vi "Text_Receiver.vi"() -> ()   [LabVIEW 2013]
uses:
  NetHackrf.dll
  <vilib>/addons/Modulation/niDMT.lvlib
panel:
  out "Symbol Rate\n[symbols/sec]":dbl=25000.0 format="%#.6p"
  in  "synchronization parameters":T1={"expected sync location (symbols)"=-1, "sync sequence"=[], "sync location uncertainty (symbols)"=0, "sync indent (symbols)"=0} {"sync sequence" format="%.2f"}
  in  "stop":bool
  in  "Tab Control":T2(tab)=enum."Rx Display"
  in  "Acquisition Duration [sec]":dbl=0.04 format="%#.6p"
  in  "Choose a PSK \nFormat":T3(tab)=enum."QPSK" caption="PSK"
  in  "BPSK System Parameters":T4={"Samples per Symbol"=8, "symbol map"=[], "Differential PSK"=enum."disable", "PSK type"=0} {"PSK type" items=["normal", "shifted", "offset"]; "symbol map" format="%.3f"}
  in  "QPSK System Parameters":T4={"Samples per Symbol"=8, "symbol map"=[], "Differential PSK"=enum."disable", "PSK type"=0} {"PSK type" items=["normal", "shifted", "offset"]; "symbol map" format="%.3f"}
  in  "pi/4 DQPSK System Parameters":T4={"Samples per Symbol"=8, "symbol map"=[], "Differential PSK"=enum."enable", "PSK type"=1} {"PSK type" items=["normal", "shifted", "offset"]; "symbol map" format="%.3f"}
  in  "OQPSK System Parameters":T4={"Samples per Symbol"=8, "symbol map"=[], "Differential PSK"=enum."disable", "PSK type"=2} {"PSK type" items=["normal", "shifted", "offset"]; "symbol map" format="%.3f"}
  in  "8-PSK System Parameters":T4={"Samples per Symbol"=8, "symbol map"=[], "Differential PSK"=enum."disable", "PSK type"=0} {"PSK type" items=["normal", "shifted", "offset"]; "symbol map" format="%.3f"}
  in  "16-PSK System Parameters":T4={"Samples per Symbol"=8, "symbol map"=[], "Differential PSK"=enum."disable", "PSK type"=0} {"PSK type" items=["normal", "shifted", "offset"]; "symbol map" format="%.3f"}
  in  "M":i32=4 min=2 step=2
  in  "Custom System Parameters":T4={"Samples per Symbol"=8, "symbol map"=[], "Differential PSK"=enum."disable", "PSK type"=0} {"PSK type" items=["normal", "shifted", "offset"]; "symbol map" format="%.3f"}
  in  "filter parameters":T5={"Alpha"=0.5, "Filter Length"=6, "TX Filter"=enum."Root Raised Cos"} caption="Matching Filter Parameters" {"Alpha" format="%.2f"}
  in  "PN Sequence Order for Sync":i32=31
  in  "Packet Parameters":T6={"Guard Bits "=30, "Sync Bits"=20, "Message Bits"=128, "Number of Packets \nto Expect"=46}
  out "Recovered Message":string
  out "Received Signal (Raw)":dbl[](graph)
  out "Constellation Graph":T7(graph)
  out "Sync Found":bool
  out "Correct Packets Rx":i16
  in  "Continuous Acquire?":bool
  out "Singal & Noise Power":cluster{"signal_power":dbl, "noise_power":dbl}={"signal_power"=1.4546950663593878e-09, "noise_power"=2.571229598792933e-12}
  out "error out":errorcluster={"status"=FALSE, "code"=1074118647, "source"="niUSRP Fetch Rx Data (CDB Cluster).vi<ERR>Overflow: an internal receive buffer has filled before the data could be returned.  Consider reducing the IQ rate, increasing the Fetch rate, or increasing the number of samples per Fetch."}
  out "Cumulative Packets Recovered":i16(graph)
  out "Signal and Noise Power Tracking":cluster{"total_power":dbl, "noise_power":dbl}(graph)={"total_power"=1.4546950663593878e-09, "noise_power"=2.571229598792933e-12}
  # "Packet Receiver"
  # "Continuous Acquire 设置为TRUE，Stop才有用"
  # "Guard\nBand"
  # "Sync\nSeq"
  # "Packet\nNumber"
  # "Pad\nData"
  # "Blank\nFrame"
  # "Data"
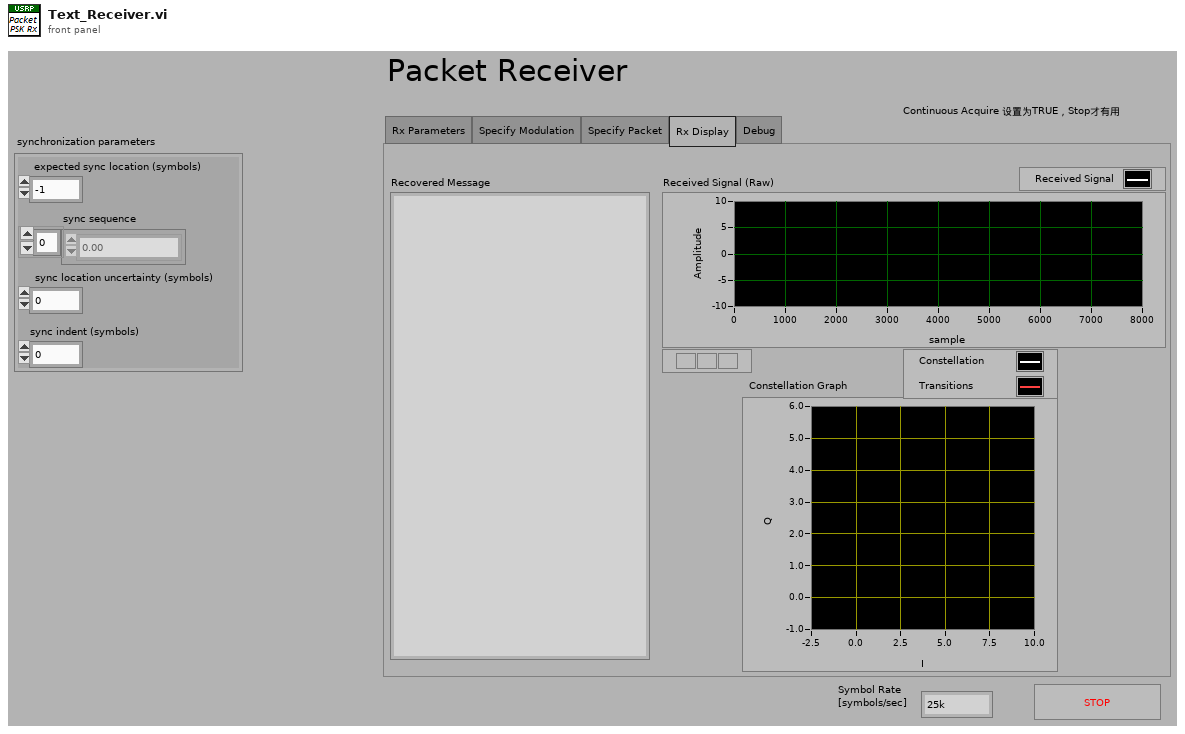
[diagram p1: front panel]
types:
  T1 = cluster{"expected sync location (symbols)":i32, "sync sequence":cdb[], "sync location uncertainty (symbols)":i32, "sync indent (symbols)":i32}
  T2 = enum32{"Rx Parameters", "Specify Modulation", "Specify Packet", "Rx Display", "Debug"}
  T3 = enum32{"BPSK", "QPSK", "pi/4DQPSK", "OQPSK", "8-PSK", "16-PSK", "Custom"}
  T4 = cluster{"Samples per Symbol":i32, "symbol map":cdb[], "Differential PSK":enum16{"disable", "enable"}, "PSK type":u16}
  T5 = cluster{"Alpha":dbl, "Filter Length":i32, "TX Filter":enum16{"none", "Raised Cosine", "Root Raised Cos", "Gaussian"}}
  T6 = cluster{"Guard Bits ":i32, "Sync Bits":i32, "Message Bits":i32, "Number of Packets \nto Expect":i32}
  T7 = cluster{"Decimated Array":dbl[], "Decimated Array":dbl[]}[]
  T8 = cluster{"Packet Array":i32[][], "IP Array of Pkt Nums Received  ":bool[]}
  T9 = cluster{"bit stream ":i8[][], "Sync Valid?":bool[], "Decoded Pkt Numbers":u32[], "Enable?":bool}
  T10 = cluster{"packet_arr":cdb[][], "Packets Valid?":bool}
  T11 = cluster{"PSK type":u16, "Samples per Symbol":i32, "Differential PSK":enum16{"disable", "enable"}, "M":i32}
  T12 = cluster{"PSK system parameters":cluster{"samples per symbol (16)":i32, "symbol map":cdb[], "differential PSK":enum16{"disable", "enable"}, "PSK type":u16}, "pulse shaping filter coefficients":dbl[], "matched filter coefficients":dbl[], "synchronization parameters":cluster{"expected sync location (symbols)":i32, "sync sequence":cdb[], "sync location uncertainty (symbols)":i32, "sync indent (symbols)":i32}, "Sync Bits":i8[]}
  T13 = typedef "niAMT.lvlib/Complex Data Waveform.ctl" = cluster{"t0":dbl, "dt":dbl, "Y":cdb[]}
  T14 = cluster{"constellation":dbl[], "oversampled data":dbl[]}[]
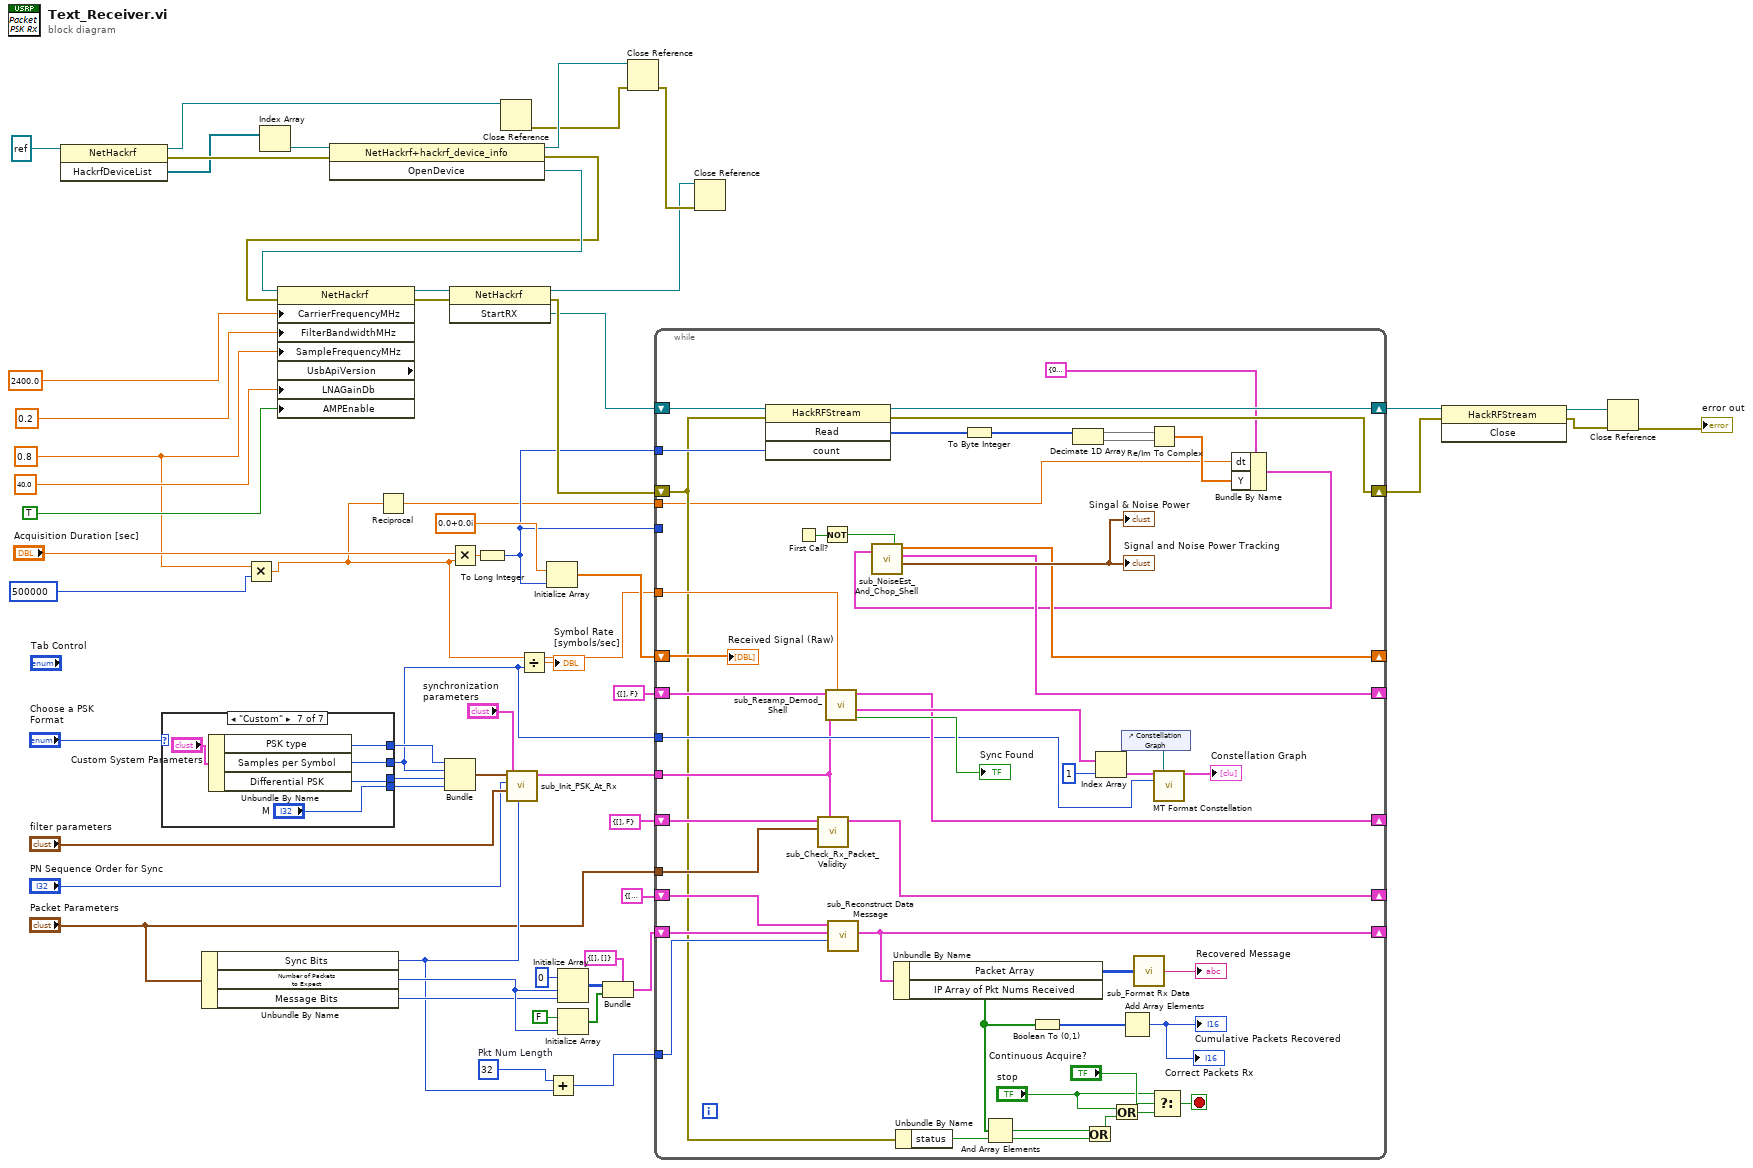
[diagram p0: block diagram]
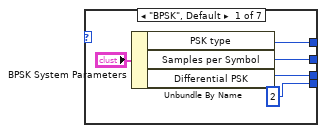
[diagram p2: hidden frame]
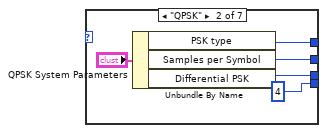
[diagram p3: hidden frame]
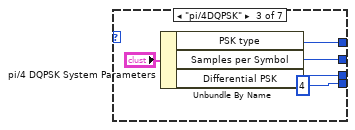
[diagram p4: hidden frame]
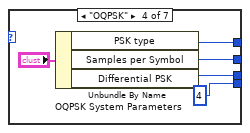
[diagram p5: hidden frame]
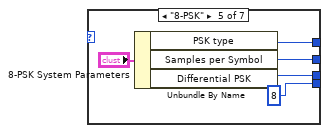
[diagram p6: hidden frame]
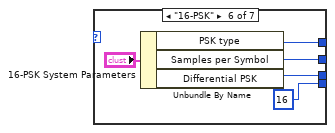
[diagram p7: hidden frame]
diagram:
  w13 = 0.8 ("SampleFrequencyMHz")
  w46 = 32  # Pkt Num Length
  n1 = invoke class="NetHackrf" method="HackrfDeviceList"(reference=refnum<k24> refnum) -> (reference out=w20:refnum<k24>, error out=w29:errorcluster, "HackrfDeviceList"=w27:refnum<k24>[])  [unwired: 2 in]
  n2 = case shown="\"Custom\"" "Choose a PSK \nFormat" {
    tunnel: [w62 w68 w73 w78 w83 w89 w92] -> w43
    tunnel: [w63 w66 w72 w77 w82 w88 w93] -> w52
    tunnel: [2 ("M-PSK (4)") 4 ("M-PSK (4)") 4 ("M-PSK (4)") 4 ("M-PSK (4)") 8 ("M-PSK (4)") 16 ("M-PSK (4)") "M"] -> w51
    tunnel: [w64 w67 w71 w76 w84 w87 w94] -> w53
    frame "BPSK", Default {
      n3 = Unbundle By Name("BPSK System Parameters") -> ("PSK type"=w64:u16, "Samples per Symbol"=w62:i32, "Differential PSK"=w63:enum16{"disable", "enable"})
    }
    frame "QPSK" {
      n4 = Unbundle By Name("QPSK System Parameters") -> ("PSK type"=w67:u16, "Samples per Symbol"=w68:i32, "Differential PSK"=w66:enum16{"disable", "enable"})
    }
    frame "pi/4DQPSK" {
      n5 = Unbundle By Name("pi/4 DQPSK System Parameters") -> ("PSK type"=w71:u16, "Samples per Symbol"=w73:i32, "Differential PSK"=w72:enum16{"disable", "enable"})
    }
    frame "OQPSK" {
      n6 = Unbundle By Name("OQPSK System Parameters") -> ("PSK type"=w76:u16, "Samples per Symbol"=w78:i32, "Differential PSK"=w77:enum16{"disable", "enable"})
    }
    frame "8-PSK" {
      n7 = Unbundle By Name("8-PSK System Parameters") -> ("PSK type"=w84:u16, "Samples per Symbol"=w83:i32, "Differential PSK"=w82:enum16{"disable", "enable"})
    }
    frame "16-PSK" {
      n8 = Unbundle By Name("16-PSK System Parameters") -> ("PSK type"=w87:u16, "Samples per Symbol"=w89:i32, "Differential PSK"=w88:enum16{"disable", "enable"})
    }
    frame "Custom" {
      n9 = Unbundle By Name("Custom System Parameters") -> ("PSK type"=w94:u16, "Samples per Symbol"=w92:i32, "Differential PSK"=w93:enum16{"disable", "enable"})
    }
  }
  n10 = Unbundle By Name("Packet Parameters") -> ("Sync Bits"=w34:i32, "Number of Packets \nto Expect"=w45:i32, "Message Bits"=w44:i32)
  n11 = Multiply(x=w13, y=500000) -> (x*y=w3:dbl)
  n12 = Index Array(array=w27) -> (element=w26:refnum<k24>)  [unwired: 1 in]
  n13 = invoke class="NetHackrf+hackrf_device_info" method="OpenDevice"(reference=w26, error in=w29) -> (reference out=w21:refnum<k24>, error out=w15:errorcluster, "OpenDevice"=w16:refnum<k24>)  [unwired: 1 in]
  n14 = property class="NetHackrf" props=["CarrierFrequencyMHz", "FilterBandwidthMHz", "SampleFrequencyMHz", "UsbApiVersion", "LNAGainDb", "AMPEnable"](reference=w16, error in=w15, "CarrierFrequencyMHz"=2400.0, "FilterBandwidthMHz"=0.2, "SampleFrequencyMHz"=w13, "LNAGainDb"=40.0, "AMPEnable"=TRUE) -> (reference out=w24:refnum<k24>, error out=w23:errorcluster)  [unwired: 1 out]
  n15 = Reciprocal(x=w3) -> (1/x=w2:dbl)
  n16 = Bundle("PSK type"=w53, "Samples per Symbol"=w43, "Differential PSK"=w52, "M"=w51) -> (w49:T11)  [unwired: 1 in]
  n17 = invoke class="NetHackrf" method="StartRX"(reference=w24, error in=w23) -> (reference out=w7:refnum<k24>, error out=w12:errorcluster, "StartRX"=w9:refnum<k24>)  [unwired: 1 in]
  n18 = Multiply(x="Acquisition Duration [sec]", y=w3) -> (x*y=w58:dbl)
  n19 = To Long Integer(number=w58) -> (32bit integer=w11:i32)
  n20 = Close Reference(reference=w20) -> (error out=w17:errorcluster)  [unwired: 1 in]
  n21 = call "sub_Init_PSK_At_Rx.vi"("Sync Bits"=w34, "synchronization parameters"="synchronization parameters", "filter parameters"="filter parameters", "PN sequence order (9)"="PN Sequence Order for Sync", "PSK Parameters"=w49) -> ("PSK Init Parameters"=w48:T12)  [unwired: 5 in, 1 out]
  n22 = Divide(x=w3, y=w43) -> (x/y=→"Symbol Rate\n[symbols/sec]":dbl)
  n23 = Initialize Array(cdb 0.0+0.0i ("element"), w11) -> (w35:cdb[])
  n24 = Add(x=w46, y=w34) -> (x+y=w54:i32)
  n25 = Initialize Array(0, w45, w44) -> (w37:i32[][])
  n26 = Initialize Array(FALSE, w45) -> (w36:bool[])
  n27 = Bundle(cluster=T8 {"Packet Array"=[], "IP Array of Pkt Nums Received  "=[]} ("Packet Info"), "Packet Array"=w37, "IP Array of Pkt Nums Received"=w36) -> (w31:T8)
  n28 = Close Reference(reference=w21, error in (no error)=w17) -> (error out=w8:errorcluster)
  n29 = while {
    tunnel: w3 -> [w143]
    tunnel: w11 -> [_]
    tunnel: "Packet Parameters" -> [w142]
    tunnel: w54 -> [w116]
    tunnel: w48 -> [w109]
    shift-right: [w103] -> w4
    shift-left: w12 -> [w104]
    tunnel: w43 -> [w110]
    shift-right: [w114] -> _
    shift-left: w31 -> [w117]
    shift-right: [w121] -> _
    shift-left: T10 {"packet_arr"=[], "Packets Valid?"=FALSE} -> [w122]
    shift-right: [w119] -> _
    shift-left: cluster{"bit stream":i8[][], "Enable?":bool} {"bit stream"=[], "Enable?"=FALSE} ("Output Bitstream") -> [w120]
    shift-right: [w108] -> _
    shift-left: T9 {"bit stream "=[], "Sync Valid?"=[], "Decoded Pkt Numbers"=[], "Enable?"=FALSE} ("Output Bit Stream") -> [w118]
    shift-right: [w111] -> _
    shift-left: w35 -> [w112]
    tunnel: w11 -> [w107]
    shift-right: [w105] -> w10
    shift-left: w9 -> [w106]
    tunnel: w2 -> [w100]
    stop <- w138 stop-if-true
    n30 = invoke class="HackRFStream" method="Read"(reference=w106, error in=w104, "count"=w107) -> (reference out=w105:refnum<k24>, error out=w103:errorcluster, "Read"=w95:u8[])  [unwired: 1 in, 1 out]
    n31 = First Call?() -> (First Call?: T/F=w128:bool)
    n32 = call "sub_Check_Rx_Packet_Validity.vi"("PSK Init Parameters"=w109, "Packet Parameters"=w142, "Input Bit Stream"=w120) -> ("Output Bit Stream"=w108:T9)  [unwired: 7 in]
    n33 = Not(x=w128) -> (.not. x?=w127:bool)
    n34 = call "sub_Resamp_Demod_Shell.vi"("Rx IQ Sampling\nRate [s/sec]"=w143, "PSK Init Parameters"=w109, "Input Packets"=w122) -> ("Synch Found?"=→"Sync Found":bool, "recovered complex waveform"=w131:T13[], "Output Bitstream"=w119:cluster{"bit stream":i8[][], "Enable?":bool})  [unwired: 3 in]
    n35 = call "sub_Reconstruct Data Message.vi"("Start Loc of Data"=w116, "Packet Info"=w117, "Input Stream"=w118) -> ("Packet Info out"=w114:T8)  [unwired: 8 in]
    n36 = Unbundle By Name(w114) -> ("Packet Array"=w115:i32[][], "IP Array of Pkt Nums Received"=w113:bool[])
    n37 = Unbundle By Name(w104) -> ("status"=w124:bool)
    n38 = To Byte Integer(number=w95) -> (8bit integer=w98:i8[])
    n39 = And Array Elements(Boolean array=w113) -> (logical AND=w125:bool)
    n40 = Boolean To (0,1)(Boolean=w113) -> (0, 1=w141:i16[])
    n41 = Decimate 1D Array(w98) -> (w97:i8[], w96:i8[])
    n42 = Or(x=w125, y=w124) -> (x .or. y?=w123:bool)
    n43 = Index Array(array=w131, index=1) -> (element=w130:T13)
    n44 = Or(x="stop", y=w123) -> (x .or. y?=w139:bool)
    n45 = control-ref of="Constellation Graph"() -> (w133:refnum<vi>)
    n46 = Add Array Elements(numeric array=w141) -> (sum=→"Correct Packets Rx" →"Cumulative Packets Recovered":i16)
    n47 = call "sub_Format Rx Data.vi"("Output Packet Array"=w115) -> ("Received Message"=→"Recovered Message":string)
    n48 = Re/Im To Complex(1:w96, 2:w97) -> (0:w101:cdb[])
    n49 = Select(t="stop", s="Continuous Acquire?", f=w139) -> (s? t:f=w138:bool)
    n50 = call <vilib>:"MT Format Constellation.vi"("waveform"=w130, "constellation reference"=w133, "samples per symbol"=w110) -> ("constellation graph"=→"Constellation Graph":T14)  [unwired: 2 in, 10 out]
    n51 = Bundle By Name(cluster=cluster{"t0":dbl, "dt":dbl, "Y":cdb[]} {"t0"=0.0, "dt"=0.0, "Y"=[]} ("s? t:f"), "dt"=w100, "Y"=w101) -> (w99:cluster{"t0":dbl, "dt":dbl, "Y":cdb[]})
    n52 = call "sub_NoiseEst_And_Chop_Shell.vi"("data"=w99, "Enable"=w127) -> ("Singal & Noise Power"=→"Signal and Noise Power Tracking" →"Singal & Noise Power":cluster{"signal_power":dbl, "noise_power":dbl}, "Output Packets"=w121:cluster{"Packets":cdb[][], "Enable?":bool}, "Delay signal (for plotting use only)"=w111:cdb[])  [unwired: 3 in]
    "Received Signal (Raw)" <- w112
  }
  n53 = Close Reference(reference=w7, error in (no error)=w8) -> ()  [unwired: 1 out]
  n54 = invoke class="HackRFStream" method="Close"(reference=w10, error in=w4) -> (reference out=w6:refnum<k24>, error out=w5:errorcluster)  [unwired: 1 in, 1 out]
  n55 = Close Reference(reference=w6, error in (no error)=w5) -> (error out=→"error out":errorcluster)
